vi "FPGA_CounterOpen.vi"   [LabVIEW 2017]
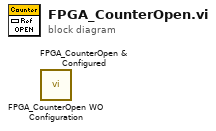
[diagram p0: block diagram]
diagram:
  n1 = call <vilib>:"FPGA_CounterOpen WO Configuration.vi"() -> ()  [unwired: 10 in, 2 out]
  n2 = call <vilib>:"FPGA_CounterOpen & Configured.vi"() -> ()  [unwired: 10 in, 2 out]
